vi "color difuso prueba.vi"() -> ()   [LabVIEW 2020]
uses:
  <vilib>/addons/Fuzzy Logic/FL Fuzzy Controller (MISO).vi
  <vilib>/addons/Fuzzy Logic/NI_Fuzzy_Logic_API.lvlib
panel:
  out "32bit integer":i32
  in  "file path":path
  in  "stop":bool
  in  "B":u8(slide) scale=0.0..255.0
  in  "G":u8(slide) scale=0.0..255.0
  in  "R":u8(slide) scale=0.0..255.0
  out "Color":u32(colorbox)
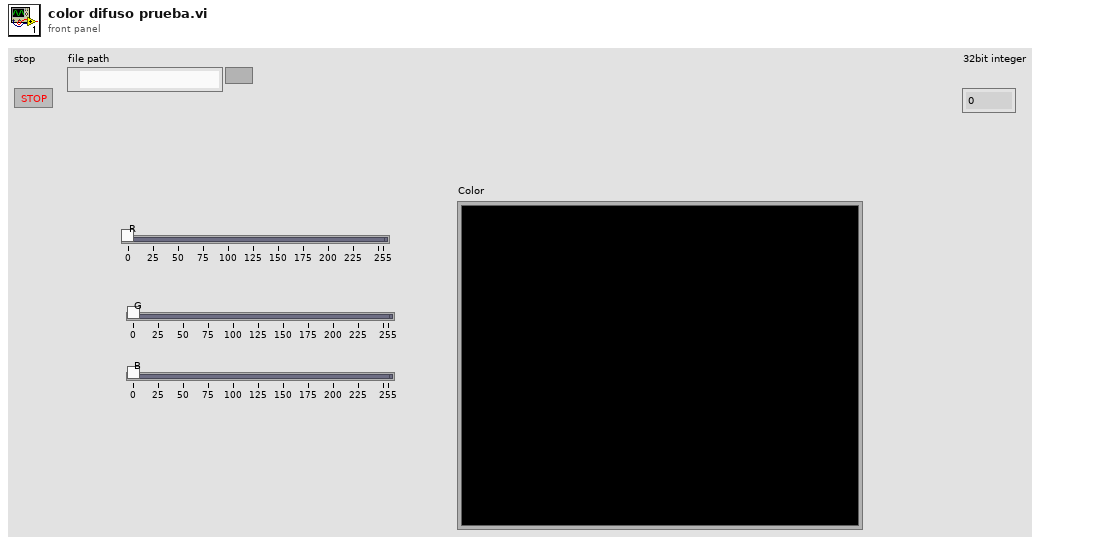
[diagram p1: front panel]
types:
  T1 = typedef "NI_Fuzzy_Logic_API.lvlib/FL System.ctl" = cluster{"input variables":T2[], "output variables":T2[], "rules":T5[], "defuzzification method":T11, "description":string, "user MF interpolating polynomials":T12[]}
  T2 = typedef "NI_Fuzzy_Logic_API.lvlib/FL Variable.ctl" = cluster{"name":string, "range":dbl[], "MFs":T3[]}
  T3 = typedef "NI_Fuzzy_Logic_API.lvlib/FL Membership Function.ctl" = cluster{"name":string, "shape":T4, "points":dbl[], "color":u32, "user-defined shape index":i32}
  T4 = typedef "NI_Fuzzy_Logic_API.lvlib/FL Membership Function Shape.ctl" = u16
  T5 = typedef "NI_Fuzzy_Logic_API.lvlib/FL Rule.ctl" = cluster{"antecedents":T6[], "antecedent connective":T8, "consequents":T9[], "consequent implication":T10, "degree of support":dbl}
  T6 = typedef "NI_Fuzzy_Logic_API.lvlib/FL Antecedent.ctl" = cluster{"Var Index":i32, "MF Index":i32, "Cond":T7}
  T7 = typedef "NI_Fuzzy_Logic_API.lvlib/FL Modifier.ctl" = u16
  T8 = typedef "NI_Fuzzy_Logic_API.lvlib/FL Antecedent Connective.ctl" = u16
  T9 = typedef "NI_Fuzzy_Logic_API.lvlib/FL Consequent.ctl" = cluster{"Var Index":i32, "MF Index":i32, "Cond":T7}
  T10 = typedef "NI_Fuzzy_Logic_API.lvlib/FL Consequent Implication.ctl" = u16
  T11 = typedef "NI_Fuzzy_Logic_API.lvlib/FL Defuzzification.ctl" = u16
  T12 = typedef "NI_Fuzzy_Logic_API.lvlib/FL Interpolating polynomials.ctl" = cluster{"X":dbl[], "Y":dbl[], "Y(x) coeff":dbl[][], "X(y) coeff":dbl[][], "Area(y) coeff":dbl[][], "coa_x(y) coeff":dbl[][]}
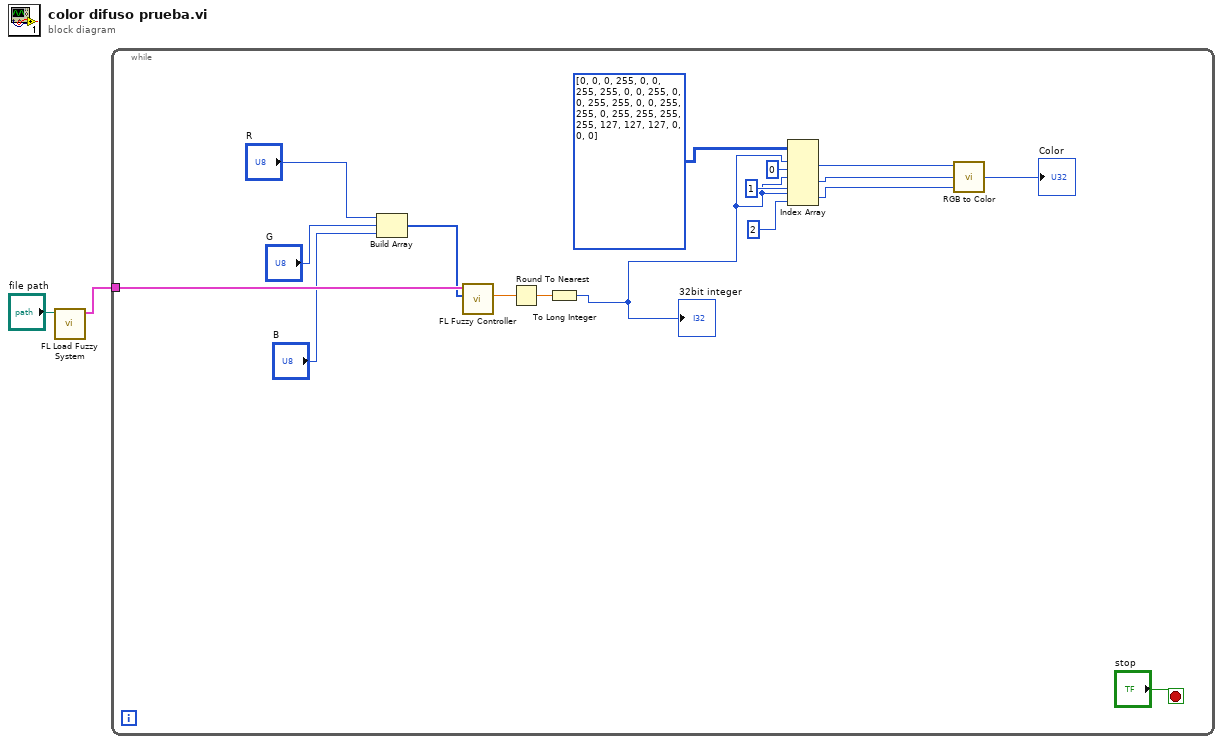
[diagram p0: block diagram]
diagram:
  n1 = call <vilib>:"FL Load Fuzzy System.vi"("file path"="file path") -> ("fuzzy system out"=w2:T1)  [unwired: 9 in, 1 out]
  n2 = while {
    tunnel: w2 -> [w17]
    stop <- "stop" stop-if-true
    n3 = Build Array("R", "G", "B") -> (w13:u8[])
    n4 = call-poly <vilib>:"FL Fuzzy Controller.vi"("input values"=w13, "fuzzy system in"=w17) -> ("output value"=w12:dbl)  [unwired: 5 in, 4 out]
    n5 = Round To Nearest(number=w12) -> (nearest integer value=w3:dbl)
    n6 = To Long Integer(number=w3) -> (32bit integer=w7:i32)
    "32bit integer" <- w7
    n7 = Index Array(array=u8[][] [[0, 0, 0], [255, 0, 0], [255, 255, 0], [0, 255, 0], [0, 255, 255], [0, 0, 255], [255, 0, 255], [255, 255, 255], [127, 127, 127], [0, 0, 0]], index (row) #1=w7, index (col) #1=0 ("disabled index (col)"), index (row) #2=w7, index (col) #2=1 ("index (col)"), index (row) #3=w7, index (col) #3=2 ("index (col)")) -> (element #1=w6:u8, element #2=w5:u8, element #3=w4:u8)
    n8 = call <vilib>:"RGB to Color.vi"("B"=w4, "G"=w5, "R"=w6) -> ("Color"=→"Color":u32)
  }
